vi "Init_Map (SubVI).vi"(8 "error in (no error)":errorcluster) -> (0 "error out":errorcluster, 3 "Probabilistic_OccupancyGrid out":refnum<class "Probabilistic_OccupancyGrid.lvclass">)   [LabVIEW 2017]
doc: "Initialise Probabilistic Map object"
uses:
  Probabilistic_map/Probabilistic_OccupancyGrid.lvclass
  Probabilistic_map/Probabilistic_OccupancyGrid.lvclass/Probabilistic_OccupancyGrid.ctl
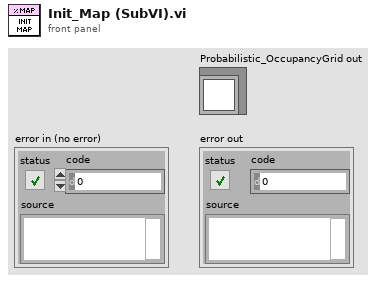
[diagram p1: front panel]
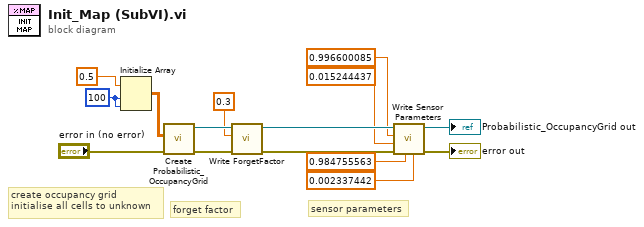
[diagram p0: block diagram]
diagram:
  w13 = 100 ("dimension size")
  # "sensor parameters"
  # "forget factor"
  # "create occupancy grid\ninitialise all cells to unknown"
  n1 = Initialize Array(0.5 ("element"), w13, w13) -> (w14:dbl[][])
  n2 = call "Create Probabilistic_OccupancyGrid.vi"("error in (no error)"="error in (no error)", "occupancy grid"=w14) -> ("error out"=w12:errorcluster, "Probabilistic_OccupancyGrid out"=w9:refnum<class "Probabilistic_OccupancyGrid.lvclass">)  [unwired: 8 in]
  n3 = call "Write ForgetFactor.vi"("error in (no error)"=w12, "ForgetFactor"=0.3 ("Map_Forget_factor"), "Probabilistic_OccupancyGrid in"=w9) -> ("error out"=w10:errorcluster, "Probabilistic_OccupancyGrid out"=w6:refnum<class "Probabilistic_OccupancyGrid.lvclass">)  [unwired: 7 in]
  n4 = call "Write Sensor Parameters.vi"("Sensor_false_positive"=0.002337442 ("log_odd_sensor_detected"), "Sensor_true_negative"=0.984755563 ("log_odd_sensor_detected"), "error in (no error)"=w10, "Sensor_false_negative"=0.015244437 ("log_odd_sensor_detected"), "Sensor_true_positive"=0.996600085 ("log_odd_sensor_detected"), "Probabilistic_OccupancyGrid in"=w6) -> ("error out"=→"error out":errorcluster, "Probabilistic_OccupancyGrid out"=→"Probabilistic_OccupancyGrid out":refnum<class "Probabilistic_OccupancyGrid.lvclass">)  [unwired: 4 in]
